vi "Compare and Append Run.vi"(8 "error in (no error)":errorcluster, 9 "Repetitions":u32, 10 "Run":refnum<class "Run Instance.lvclass">, 11 "Optimiser Cell in":refnum<class "Optimiser Cell.lvclass">) -> (0 "error out":errorcluster, 1 "Cell Updated":bool, 2 "new Schedule Cell out":refnum<class "Schedule Cell.lvclass">, 3 "Optimiser Cell out":refnum<class "Optimiser Cell.lvclass">)   [LabVIEW 2020, in "TALOS.lvlib" / "Run Utilities.lvlib" / "Optimiser Cell.lvclass"]
doc: "VI compares the Run Instance with the Cell. If they are the same, it increases the number of repetitions. Otherwise, it creates a new Cell"
uses:
  Optimiser Cell.lvclass
  C:/LabVIEW Code/TALOS/talos/Run Utilities/Cell/Schedule Cell.lvclass
  Run Instance/Run Instance.lvclass
  Cell/Schedule Cell.lvclass
  Optimiser Cell.lvclass/Optimiser Cell.ctl
  Run Utilities.lvlib
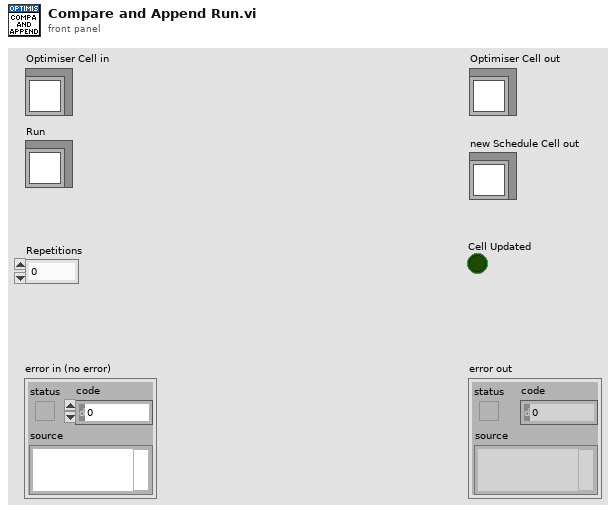
[diagram p1: front panel]
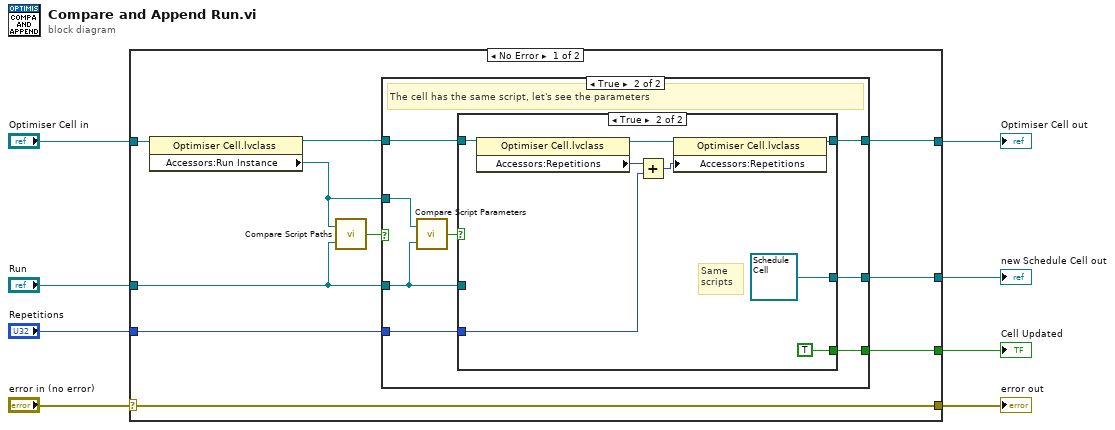
[diagram p0: block diagram]
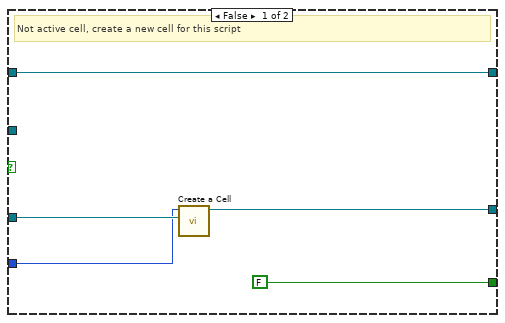
[diagram p2: hidden frame]
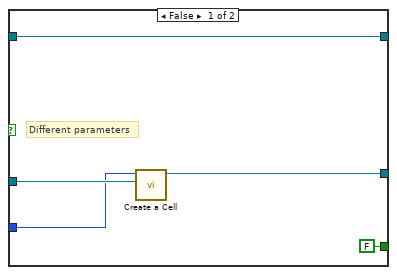
[diagram p3: hidden frame]
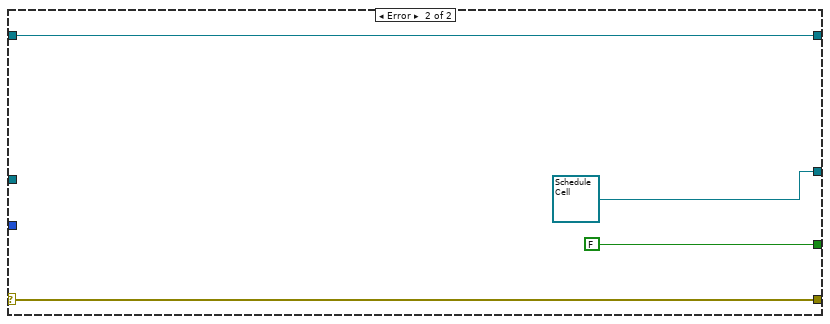
[diagram p4: hidden frame]
diagram:
  n1 = case shown="No Error" "error in (no error)" {
    selector: "error in (no error)" -> [w18 w48]
    tunnel: [w18 w48] -> w5
    tunnel: [w10 w47] -> w7
    tunnel: "Optimiser Cell in" -> [w17 w47]
    tunnel: "Run" -> [w13 _]
    tunnel: "Repetitions" -> [w15 _]
    tunnel: [w9 refnum<class "Schedule Cell.lvclass"> refnum ("Schedule Cell out")] -> w6
    tunnel: [w16 FALSE] -> w4
    frame No Error {
      n2 = property class="Optimiser Cell.lvclass"(reference=w17) -> (reference out=w11:refnum<class "Optimiser Cell.lvclass">, "Accessors:Run Instance"=w12:refnum<class "Run Instance.lvclass">)  [unwired: 1 in, 1 out]
      n3 = call "Compare Script Paths.vi"("Run Instance B"=w13, "Run Instance A"=w12) -> ("Same?"=w14:bool)
      n4 = case shown="True" w14 {
        tunnel: [w23 w31] -> w9
        tunnel: [FALSE ("Optimiser") w30] -> w16
        tunnel: w13 -> [w22 w28]
        tunnel: w15 -> [w20 w29]
        tunnel: w12 -> [_ w27]
        tunnel: w11 -> [w19 w25]
        tunnel: [w19 w24] -> w10
        frame False {
          # "Not active cell, create a new cell for this script"
          n5 = call "Create a Cell.vi"("Run Instance"=w22, "Repetitions"=w20) -> ("Schedule Cell out"=w23:refnum<class "Schedule Cell.lvclass">)  [unwired: 8 in, 1 out]
        }
        frame True {
          # "The cell has the same script, let's see the parameters"
          n6 = call "Compare Script Parameters.vi"("Run Instance B"=w28, "Run Instance A"=w27) -> ("Same?"=w26:bool)
          n7 = case shown="True" w26 {
            tunnel: w28 -> [w36 _]
            tunnel: [w35 refnum<class "Schedule Cell.lvclass"> refnum ("Schedule Cell out")] -> w31
            tunnel: [FALSE ("Optimiser") TRUE] -> w30
            tunnel: w29 -> [w33 w38]
            tunnel: w25 -> [w32 w42]
            tunnel: [w32 w41] -> w24
            frame False {
              # "Different parameters"
              n8 = call "Create a Cell.vi"("Run Instance"=w36, "Repetitions"=w33) -> ("Schedule Cell out"=w35:refnum<class "Schedule Cell.lvclass">)  [unwired: 8 in, 1 out]
            }
            frame True {
              # "Same scripts"
              n9 = property class="Optimiser Cell.lvclass"(reference=w42) -> (reference out=w40:refnum<class "Optimiser Cell.lvclass">, "Accessors:Repetitions"=w39:u32)  [unwired: 1 in, 1 out]
              n10 = Add(x=w39, y=w38) -> (x+y=w37:u32)
              n11 = property class="Optimiser Cell.lvclass"(reference=w40, "Accessors:Repetitions"=w37) -> (reference out=w41:refnum<class "Optimiser Cell.lvclass">)  [unwired: 1 in, 1 out]
            }
          }
        }
      }
    }
    frame Error {
    }
  }
  "error out" <- w5
  "Optimiser Cell out" <- w7
  "new Schedule Cell out" <- w6
  "Cell Updated" <- w4
